vi "ExtractData.vi"(7 "Window settings":T3={"Window length (s)"=0.0, "Window step (s)"=0.0, "Window type"=1} {"Window type" items=["Rectangle"=0, "Hanning"=1, "Hamming"=2, "Blackman-Harris"=3, "Exact Blackman"=4, "Blackman"=5, "Flat Top"=6, "4 Term B-Harris "=7, "7 Term B-Harris"=8, "Low Sidelobe"=9, "Blackman Nuttall"=11, "Triangle"=30, "Bartlett-Hanning"=31, "Bohman"=32, "Parzen"=33, "Welch"=34, "Kaiser"=60, "Dolph-Chebyshev"=61, "Gaussian"=62]}, 8 "Output setup":T1, 9 "Sampling frequency":dbl, 10 "Frequency (f0)":dbl, 11 "Signal in":waveform(dbl)) -> (1 "Selected harmonics":cluster{"Amplitudes":dbl[], "Frequencies":dbl[]}, 2 "Harmonics":cluster{"Amplitudes":dbl[], "Frequencies":dbl[]}, 3 "Spectrum":cluster{"f0":dbl, "df":dbl, dbl[]})   [LabVIEW 2019]
uses:
  <vilib>/Analysis/4window.llb/windowTd.ctl
  <vilib>/measure/maspectr.llb/FFT Spectrum (Mag-Phase) for 1 Chan.vi
  <vilib>/measure/matone.llb/Extract Single Tone Information 1 Chan.vi
  <vilib>/measure/NI_MAPro.lvlib
  <vilib>/Analysis/NI_AALPro.lvlib
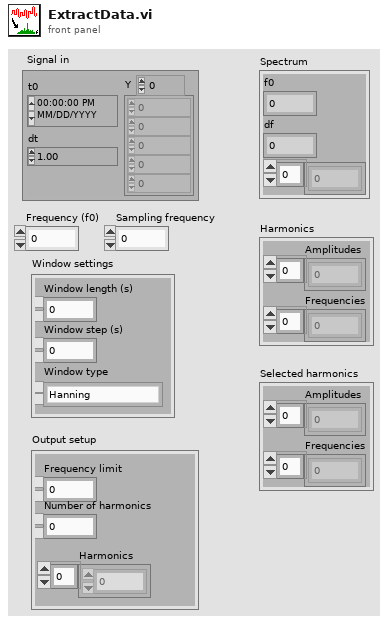
[diagram p1: front panel]
types:
  T1 = cluster{"Frequency limit":dbl, "Number of harmonics":i32, "Harmonics":i32[]}
  T2 = typedef "NI_AALPro.lvlib/windowTd.ctl" = u32
  T3 = cluster{"Window length (s)":dbl, "Window step (s)":dbl, "Window type":T2}
  T4 = enum32{"none", "input signal", "detected signal", "residual signal"}
  T5 = cluster{"approx freq. (optional)":dbl, "search (+/- % of Fsampl.)":dbl}
  T6 = cluster{"averaging mode":enum16{"No averaging", "Vector averaging", "RMS averaging", "Peak hold"}, "weighting mode":enum16{"Linear", "Exponential"}, "number of averages":u32}
  T7 = enum16{"No averaging", "Vector averaging", "RMS averaging", "Peak hold"}
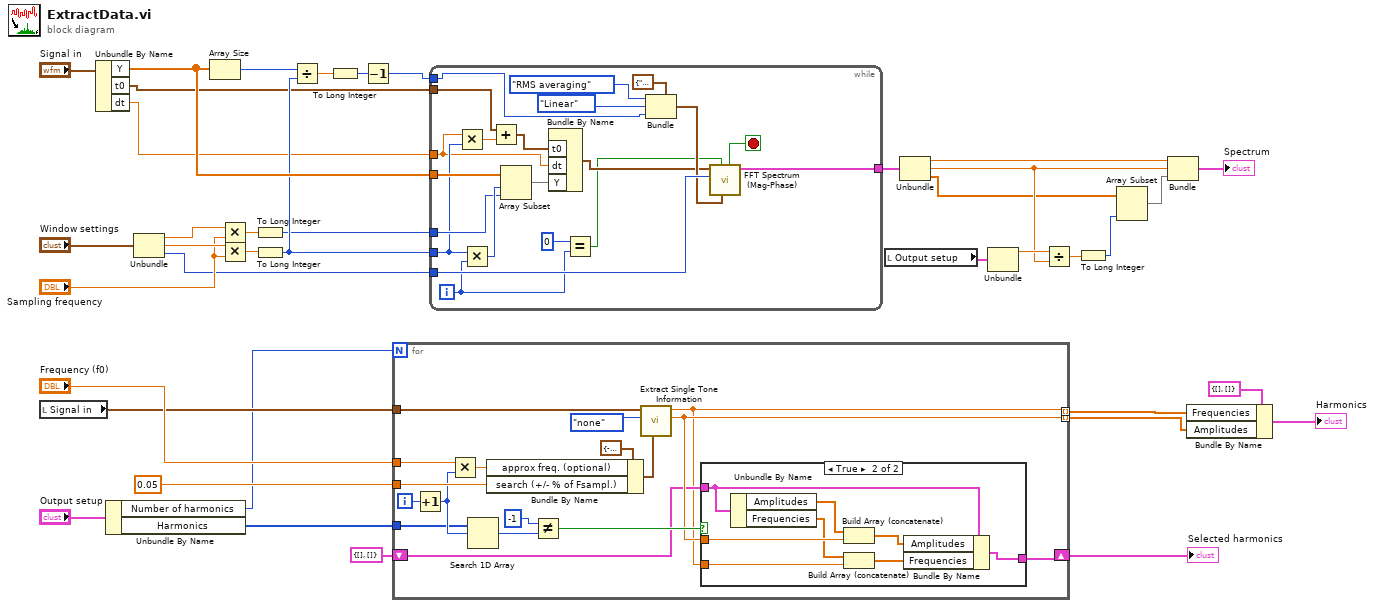
[diagram p0: block diagram]
diagram:
  n1 = local read "Signal in"() -> (w37:waveform(dbl))
  n2 = Unbundle By Name("Signal in") -> ("Y"=w24:dbl[], "t0"=w5:timestamp, "dt"=w6:dbl)
  n3 = Unbundle By Name("Output setup") -> ("Number of harmonics"=w33:i32, "Harmonics"=w34:i32[])
  n4 = Unbundle("Window settings") -> ("Window length (s)"=w31:dbl, "Window step (s)"=w30:dbl, "Window type"=w21:T2)
  n5 = Array Size(array=w24) -> (size(s)=w26:i32)
  n6 = Multiply(x=w31, y="Sampling frequency") -> (x*y=w28:dbl)
  n7 = Multiply(x=w30, y="Sampling frequency") -> (x*y=w27:dbl)
  n8 = To Long Integer(number=w28) -> (32bit integer=w22:i32)
  n9 = To Long Integer(number=w27) -> (32bit integer=w23:i32)
  n10 = Divide(x=w26, y=w23) -> (x/y=w25:dbl)
  n11 = To Long Integer(number=w25) -> (32bit integer=w2:i32)
  n12 = Decrement(x=w2) -> (x-1=w1:i32)
  n13 = for {
    N: w33 -> [_]
    tunnel: "Frequency (f0)" -> [w50]
    tunnel: 0.05 ("search (+/- % of Fsampl.)") -> [w54]
    tunnel: w37 -> [w55]
    tunnel: [w44] -> w16 mode=indexing
    shift-right: [w42] -> w18
    shift-left: cluster{"Amplitudes":dbl[], "Frequencies":dbl[]} {"Amplitudes"=[], "Frequencies"=[]} -> [w43]
    tunnel: w34 -> [w41]
    tunnel: [w40] -> w17 mode=indexing
    i -> [w56]
    n14 = Increment(x=w56) -> (x+1=w48:i32)
    n15 = Multiply(x=w50, y=w48) -> (x*y=w49:dbl)
    n16 = Search 1D Array(1D array=w41, element=w48) -> (index of element=w47:i32)  [unwired: 1 in]
    n17 = Bundle By Name(cluster=T5 {"approx freq. (optional)"=-1.0, "search (+/- % of Fsampl.)"=5.0} ("advanced search"), "approx freq. (optional)"=w49, "search (+/- % of Fsampl.)"=w54) -> (w52:T5)
    n18 = Not Equal?(x=-1, y=w47) -> (x != y?=w45:bool)
    n19 = call-poly <vilib>:"Extract Single Tone Information.vi"("advanced search"=w52, "export mode"=T4."none", "time signal in"=w55) -> ("detected amplitude"=w44:dbl, "detected frequency"=w40:dbl)  [unwired: 3 in, 4 out]
    n20 = case shown="True" w45 {
      tunnel: w44 -> [_ w65]
      tunnel: w43 -> [w57 w63]
      tunnel: [w57 w62] -> w42
      tunnel: w40 -> [_ w58]
      frame False {
      }
      frame True {
        n21 = Unbundle By Name(w63) -> ("Amplitudes"=w64:dbl[], "Frequencies"=w60:dbl[])
        n22 = Build Array (concatenate)(w64, w65) -> (w61:dbl[])
        n23 = Build Array (concatenate)(w60, w58) -> (w59:dbl[])
        n24 = Bundle By Name(cluster=w63, "Amplitudes"=w61, "Frequencies"=w59) -> (w62:cluster{"Amplitudes":dbl[], "Frequencies":dbl[]})
      }
    }
  }
  "Selected harmonics" <- w18
  n25 = while {
    tunnel: w24 -> [w86]
    tunnel: w6 -> [w75]
    tunnel: w23 -> [w76]
    tunnel: w22 -> [w84]
    tunnel: w21 -> [w82]
    tunnel: [w77] -> w4
    tunnel: w5 -> [w73]
    tunnel: w1 -> [w70]
    i -> [w69]
    stop <- w66 stop-if-true
    n26 = Multiply(x=w75, y=w76) -> (x*y=w74:dbl)
    n27 = Multiply(x=w76, y=w69) -> (x*y=w85:i32)
    n28 = Add(x=w73, y=w74) -> (x+y=w72:timestamp)
    n29 = Array Subset(array=w86, index=w85, length=w84) -> (w83:dbl[])
    n30 = Bundle By Name("t0"=w72, "dt"=w75, "Y"=w83) -> (w71:waveform(dbl))  [unwired: 1 in]
    n31 = Equal?(x=0, y=w69) -> (x = y?=w67:bool)
    n32 = Bundle(cluster=T6 {"averaging mode"=enum."No averaging", "weighting mode"=enum."Exponential", "number of averages"=10} ("averaging parameters"), "averaging mode"=T7."RMS averaging", "weighting mode"=enum16{"Linear", "Exponential"}."Linear", "number of averages"=w70) -> (w78:T6)
    n33 = call-poly <vilib>:"FFT Spectrum (Mag-Phase).vi"("averaging parameters"=w78, "restart averaging (F)"=w67, "window"=w82, "time signal"=w71) -> ("magnitude"=w77:cluster{"f0":dbl, "df":dbl, "magnitude":dbl[]}, "averaging done"=w66:bool)  [unwired: 3 in, 3 out]
  }
  n34 = local read "Output setup"() -> (w10:T1)
  n35 = Unbundle(w4) -> ("f0"=w36:dbl, "df"=w8:dbl, "magnitude"=w3:dbl[])
  n36 = Unbundle(w10) -> ("Frequency limit"=w9:dbl)  [unwired: 2 out]
  n37 = Divide(x=w9, y=w8) -> (x/y=w12:dbl)
  n38 = To Long Integer(number=w12) -> (32bit integer=w11:i32)
  n39 = Array Subset(array=w3, length=w11) -> (w13:dbl[])  [unwired: 1 in]
  n40 = Bundle("f0"=w36, "df"=w8, w13) -> (→"Spectrum":cluster{"f0":dbl, "df":dbl, dbl[]})  [unwired: 1 in]
  n41 = Bundle By Name(cluster=cluster{"Amplitudes":dbl[], "Frequencies":dbl[]} {"Amplitudes"=[], "Frequencies"=[]}, "Frequencies"=w17, "Amplitudes"=w16) -> (→"Harmonics":cluster{"Amplitudes":dbl[], "Frequencies":dbl[]})
